vi "Set Access Type.vi"(8 "error in":errorcluster, 10 "Access Type":T1, 11 "Object Entry in":refnum<class "Object Entry.lvclass">) -> (0 "error out":errorcluster, 3 "Object Entry out":refnum<class "Object Entry.lvclass">)   [LabVIEW 2020, in "CANopen.lvlib" / "Object Entry.lvclass"]
doc: "Sets access type."
uses:
  Object Entry.lvclass
  Object Entry.lvclass/Object Entry.ctl
  Sub Objects Dictionary/Sub Objects Dictionary.lvclass
  Sub Object/Sub Object.lvclass
  Typedefs/Access Type.ctl
  CANopen.lvlib
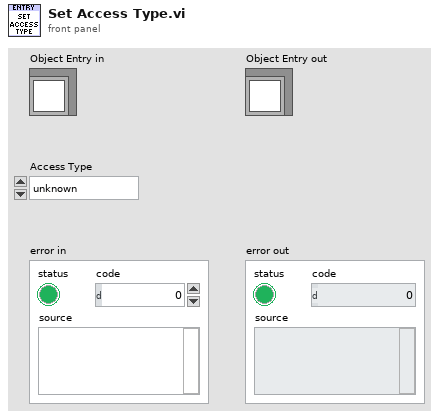
[diagram p1: front panel]
types:
  T1 = typedef "CANopen.lvlib/Access Type.ctl" = enum16{"unknown", "ro", "wo", "rw", "rwr", "rww", "const"}
  T2 = typedef "CANopen.lvlib/Object Type.ctl" = u8
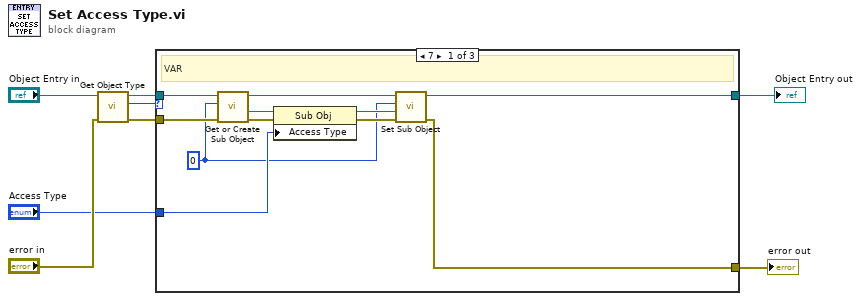
[diagram p0: block diagram]
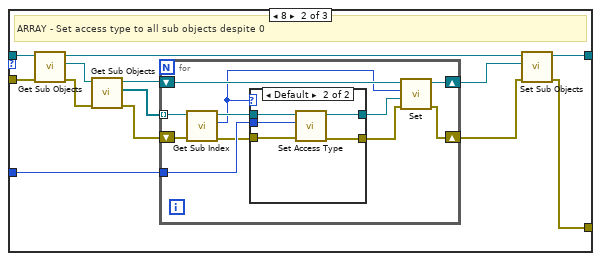
[diagram p2: hidden frame]
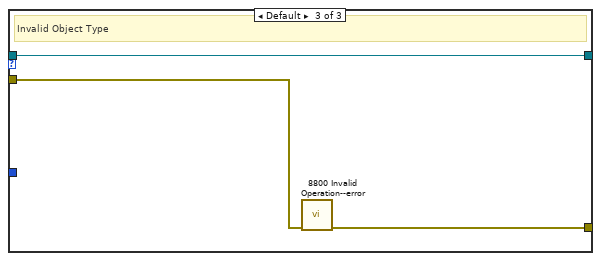
[diagram p4: hidden frame]
diagram:
  n1 = call "Get Object Type.vi"("error in"="error in", "Object Entry in"="Object Entry in") -> ("error out"=w3:errorcluster, "Object Type"=w6:T2, "Object Entry out"=w5:refnum<class "Object Entry.lvclass">)  [unwired: 7 in]
  n2 = case shown="7" w6 {
    tunnel: w5 -> [w19 w30 w51]
    tunnel: "Access Type" -> [w16 w27 _]
    tunnel: w3 -> [w15 w32 w53]
    tunnel: [w11 w20 w52] -> w2
    tunnel: [w10 w23 w51] -> w1
    frame 7 {
      w9 = u8 0 ("Sub Index")
      # "VAR"
      n3 = call "Get or Create Sub Object.vi"("error in"=w15, "Sub Index"=w9, "Obj Entry in"=w19) -> ("error out"=w18:errorcluster, "Sub Object"=w17:refnum<class "Sub Object.lvclass">, "Obj Entry out"=w14:refnum<class "Object Entry.lvclass">)  [unwired: 6 in]
      n4 = property class="Sub Obj"(reference=w17, error in=w18, "Access Type"=w16) -> (reference out=w13:refnum<class "Sub Object.lvclass">, error out=w12:errorcluster)
      n5 = call "Set Sub Object.vi"("error in"=w12, "Sub Object"=w13, "Sub Index"=w9, "Obj Entry in"=w14) -> ("error out"=w11:errorcluster, "Obj Entry out"=w10:refnum<class "Object Entry.lvclass">)  [unwired: 6 in]
    }
    frame 8 {
      # "ARRAY - Set access type to all sub objects despite 0"
      n6 = call "Get Sub Objects.vi"("error in"=w32, "Object Entry in"=w30) -> ("error out"=w31:errorcluster, "Sub Objects"=w29:refnum<class "Sub Objects Dictionary.lvclass">, "Object Entry out"=w22:refnum<class "Object Entry.lvclass">)  [unwired: 7 in]
      n7 = call "Get Sub Objects.vi"("error in (no error)"=w31, "Sub Objects Dictionary in"=w29) -> ("error out"=w28:errorcluster, "Sub Objects"=w26:refnum<class "Sub Object.lvclass">[], "Sub Objects Dictionary out"=w25:refnum<class "Sub Objects Dictionary.lvclass">)  [unwired: 7 in]
      n8 = for {
        tunnel: w26 -> [w35] mode=indexing
        tunnel: w27 -> [w42]
        shift-right: [w40] -> w24
        shift-left: w25 -> [w41]
        shift-right: [w39] -> w21
        shift-left: w28 -> [w43]
        n9 = call "Get Sub Index.vi"("error in"=w43, "Sub Object in"=w35) -> ("error out"=w36:errorcluster, "Sub Index"=w33:u8, "Sub Object out"=w34:refnum<class "Sub Object.lvclass">)  [unwired: 7 in]
        n10 = case shown="Default" w33 {
          tunnel: w34 -> [w45 w50]
          tunnel: w36 -> [w44 w49]
          tunnel: w42 -> [_ w48]
          tunnel: [w45 w47] -> w37
          tunnel: [w44 w46] -> w38
          frame 0 {
          }
          frame Default {
            n11 = call "Set Access Type.vi"("error in (no error)"=w49, "Access Type"=w48, "Sub Object in"=w50) -> ("error out"=w46:errorcluster, "Sub Object out"=w47:refnum<class "Sub Object.lvclass">)  [unwired: 7 in]
          }
        }
        n12 = call "Set.vi"("error in"=w38, "Sub Object"=w37, "Sub Index"=w33, "Sub Objects Dictionary in"=w41) -> ("error out"=w39:errorcluster, "Sub Objects Dictionary out"=w40:refnum<class "Sub Objects Dictionary.lvclass">)  [unwired: 6 in]
      }
      n13 = call "Set Sub Objects.vi"("error in (no error)"=w21, "Sub Objects Dictionary"=w24, "Object Entry in"=w22) -> ("error out"=w20:errorcluster, "Object Entry out"=w23:refnum<class "Object Entry.lvclass">)  [unwired: 7 in]
    }
    frame Default {
      # "Invalid Object Type"
      n14 = call "8800 Invalid Operation--error.vi"("error in"=w53) -> ("error out"=w52:errorcluster)  [unwired: 9 in, 1 out]
    }
  }
  "error out" <- w2
  "Object Entry out" <- w1
